vi "Brake-Activate.vi"(8 "error in (no error)":errorcluster, 11 "Motor-Maxon in":refnum<class "Motor-Maxon.lvclass">) -> (0 "error out":errorcluster, 3 "Motor-Maxon out":refnum<class "Motor-Maxon.lvclass">)   [LabVIEW 2013, in "PowderDeposition.lvlib" / "Motor-Maxon.lvclass"]
uses:
  Motor-Maxon.lvclass
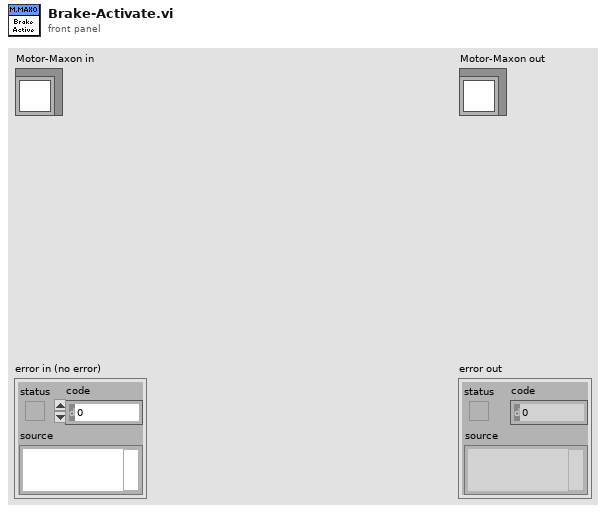
[diagram p1: front panel]
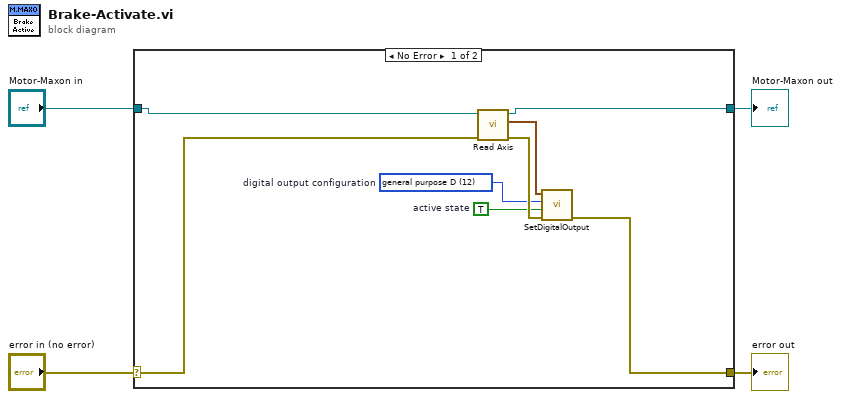
[diagram p0: block diagram]
diagram:
  n1 = case shown="No Error" "error in (no error)" {
    selector: "error in (no error)" -> [w7 w14]
    tunnel: [w6 w14] -> w3
    tunnel: [w5 w13] -> w1
    tunnel: "Motor-Maxon in" -> [w12 w13]
    frame No Error {
      w8 = u16 12 items=["ready/fault"=0, "position compare"=1, "general purpose A"=15, "general purpose B"=14, "general purpose C"=13, "general purpose D"=12, "general purpose E"=11, "general purpose F"=10, "general purpose G"=9, "general purpose H"=8]  # digital output configuration
      w9 = TRUE  # active state
      n2 = call-dynamic "Read Axis.vi"("error in (no error)"=w7, "Motor-Maxon in"=w12) -> ("error out"=w10:errorcluster, "Axis"=w11:cluster{"keyHandle":u32, "nodeID":u16}, "Motor-Maxon out"=w5:refnum<class "Motor-Maxon.lvclass">)  [unwired: 7 in]
      n3 = call <instrlib>:"SetDigitalOutput.vi"("error in (no error)"=w10, "active state"=w9, "digital output configuration"=w8, "axis in"=w11) -> ("error out"=w6:errorcluster)  [unwired: 2 in, 1 out]
    }
    frame Error {
    }
  }
  "error out" <- w3
  "Motor-Maxon out" <- w1
